vi "niRFUtil MT Add AWGN.vi"(0 "Waveform In":T1={"x0"=0.0, "dx"=1.0, "y"=[]} caption="input complex waveform" {"y" format="%.2f"; "dx" format="%^.2e"; "x0" format="%^.2e"}, 5 "samples per symbol (16)":i32=16, 7 "bits per symbol (1)":i32=1, 9 "Eb/N0 (10 dB)":dbl=10.0 format="%.2f", 11 "error in (no error)":errorcluster, 12 "seed in (0xFFFFFFFF)":i32=-1 format="%.0x", 13 "reset? (T)":bool=TRUE) -> (4 "Waveform Out":T1 caption="output complex waveform" {"y" format="%.2f"; "dx" format="%^.2e"; "x0" format="%^.2e"}, 10 "seed out":i32 format="%.0x", 15 "error out":errorcluster)   [LabVIEW 2015, in "niRFUtil.lvlib"]
doc: "Generates zero-mean complex additive white Gaussian noise (AWGN) with uniform power spectral density and adds it to the complex baseband modulated waveform."
uses:
  niRFUtil.lvlib
  Includes/niRFUtil INC Complex Waveform.ctl
  Includes/niRFUtil INC Complex Array.ctl
  <vilib>/Analysis/NI_AALBase.lvlib
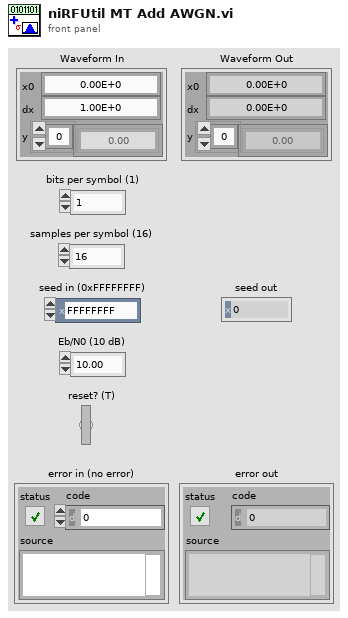
[diagram p1: front panel]
types:
  T1 = typedef "niRFUtil.lvlib/niRFUtil INC Complex Waveform.ctl" = cluster{"x0":dbl, "dx":dbl, "y":T2}
  T2 = typedef "niRFUtil.lvlib/niRFUtil INC Complex Array.ctl" = csg[]
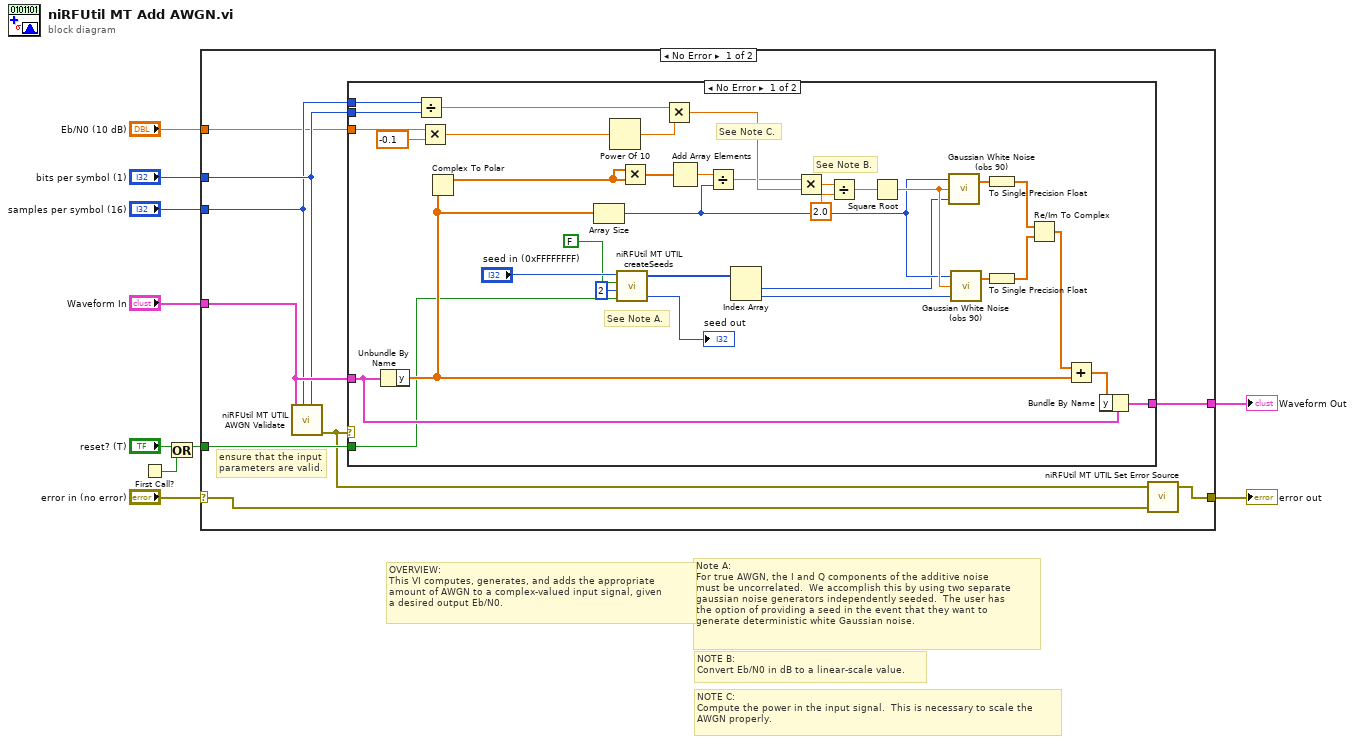
[diagram p0: block diagram]
diagram:
  # "NOTE C:\nCompute the power in the input signal.  This is necessary to scale the\nAWGN properly."
  # "NOTE B:\nConvert Eb/N0 in dB to a linear-scale value."
  # "OVERVIEW:\nThis VI computes, generates, and adds the appropriate\namount of AWGN to a complex-valued input signal, given\na desired output Eb/N0."
  # "Note A:\nFor true AWGN, the I and Q components of the additive noise\nmust be uncorrelated.  We accomplish this by using two separate\ngaussian noise generators independently seeded.  The user has\nthe option of providing a seed in the event that they want to\ngenerate deterministic white Gaussian noise."
  n1 = First Call?() -> (First Call?: T/F=w1:bool)
  n2 = Or(x="reset? (T)", y=w1) -> (x .or. y?=w2:bool)
  n3 = case shown="No Error" "error in (no error)" {
    selector: "error in (no error)" -> [w11 w55]
    tunnel: "Waveform In" -> [w19 _]
    tunnel: "bits per symbol (1)" -> [w17 _]
    tunnel: "samples per symbol (16)" -> [w16 _]
    tunnel: w2 -> [w18 _]
    tunnel: "Eb/N0 (10 dB)" -> [w15 _]
    tunnel: [w14 _] -> w5
    tunnel: [w13 w55] -> w4
    frame No Error {
      # "ensure that the input parameters are valid."
      n4 = call "niRFUtil MT UTIL AWGN Validate.vi"("Bits Per Symbol (1)"=w17, "Samples Per Symbol (16)"=w16, "Waveform In"=w19) -> ("error out"=w12:errorcluster)  [unwired: 1 in, 7 out]
      n5 = case shown="No Error" w12 {
        tunnel: w19 -> [w34 w54]
        tunnel: w18 -> [w28 _]
        tunnel: w17 -> [w42 _]
        tunnel: w16 -> [w41 _]
        tunnel: w15 -> [w39 _]
        tunnel: [w32 w54] -> w14
        frame No Error {
          # "See Note A."
          # "See Note B."
          # "See Note C."
          n6 = Unbundle By Name(w34) -> ("y"=w35:T2)
          n7 = Divide(x=w41, y=w42) -> (x/y=w44:dbl)
          n8 = Multiply(x=w39, y=-0.1) -> (x*y=w38:dbl)
          n9 = Complex To Polar(r * e^(i*theta)=w35) -> (r=w31:sgl[])  [unwired: 1 out]
          n10 = Array Size(array=w35) -> (size(s)=w47:i32)
          n11 = Power Of 10(x=w38) -> (10^x=w37:dbl)
          n12 = call "niRFUtil MT UTIL createSeeds.vi"("Reset? (T)"=w28, "# of seeds to create"=2, "Allow Neg if not already? (T)"=FALSE, "seed in (0xFFFFFFFF)"="seed in (0xFFFFFFFF)") -> ("Next seed"=→"seed out":i32, "Seeds"=w26:i32[])  [unwired: 1 out]
          n13 = Multiply(x=w31, y=w31) -> (x*y=w30:sgl[])
          n14 = Multiply(x=w44, y=w37) -> (x*y=w45:dbl)
          n15 = Add Array Elements(numeric array=w30) -> (sum=w43:sgl)
          n16 = Divide(x=w43, y=w47) -> (x/y=w36:sgl)
          n17 = Index Array(array=w26) -> (element #1=w24:i32, element #2=w25:i32)  [unwired: 2 in]
          n18 = Multiply(x=w36, y=w45) -> (x*y=w53:dbl)
          n19 = Divide(x=w53, y=2.0) -> (x/y=w51:dbl)
          n20 = Square Root(x=w51) -> (sqrt(x)=w50:dbl)
          n21 = call <vilib>:"Gaussian White Noise (obs 90).vi"("seed"=w24, "standard deviation"=w50, "samples"=w47) -> ("Gaussian noise pattern"=w48:dbl[])  [unwired: 1 out]
          n22 = call <vilib>:"Gaussian White Noise (obs 90).vi"("seed"=w25, "standard deviation"=w50, "samples"=w47) -> ("Gaussian noise pattern"=w49:dbl[])  [unwired: 1 out]
          n23 = To Single Precision Float(number=w48) -> (single precision float=w21:sgl[])
          n24 = To Single Precision Float(number=w49) -> (single precision float=w20:sgl[])
          n25 = Re/Im To Complex(1:w20, 2:w21) -> (0:w52:csg[])
          n26 = Add(x=w52, y=w35) -> (x+y=w33:T2)
          n27 = Bundle By Name(cluster=w34, "y"=w33) -> (w32:T1)
        }
        frame Error {
        }
      }
      n28 = call "niRFUtil MT UTIL Set Error Source.vi"("initial error in (no error)"=w11, "final error in (no error)"=w12) -> ("error out"=w13:errorcluster)  [unwired: 3 in]
    }
    frame Error {
    }
  }
  "error out" <- w4
  "Waveform Out" <- w5
